vi "variantCtrlString.vi"(4 "isRequired (T)":bool=TRUE, 6 "menu in (get)":enum16{"get", "set"}(ring), 8 "error in":errorcluster, 9 "String Value":string, 10 "name in":string, 11 "Step in":variant) -> (0 "error out":errorcluster, 1 "String Value":string, 2 "isFound?":bool, 3 "Step out":variant)   [LabVIEW 2024]
uses:
  controls/typeEngErrorCodes.ctl
  controls/typeStepVarients.ctl
  controls/typeProcVarientName.ctl
panel:
  out "spreadsheet string":string
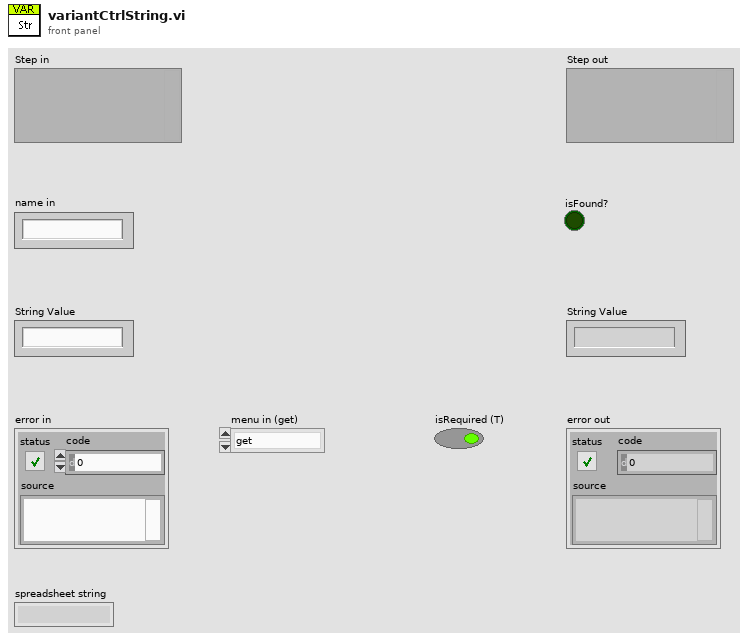
[diagram p1: front panel]
types:
  T1 = typedef "typeEngErrorCodes.ctl" = u16
  T2 = typedef "typeProcVarientName.ctl" = enum16{"procNameID", "procModuleID", "procPath", "procIsRunning", "procIndex", "procModule", "procRegisterNumeric", "procRegisterString", "procReport", "procReportPrev", "procCLK", "procStepPointer", "procType"}
  T3 = typedef "typeStepVarients.ctl" = enum16{"stepNameID", "stepFunction", "stepReport", "stepSetpoint", "stepPointer", "stepProcPointer", "stepIoPointer", "stepIoValue", "stepFilePointer", "stepMessage", "stepTimeString", "stepNumReg", "stepStrReg", "stepSeconds", "stepUnitDoseParams", "stepUnitIndex"}
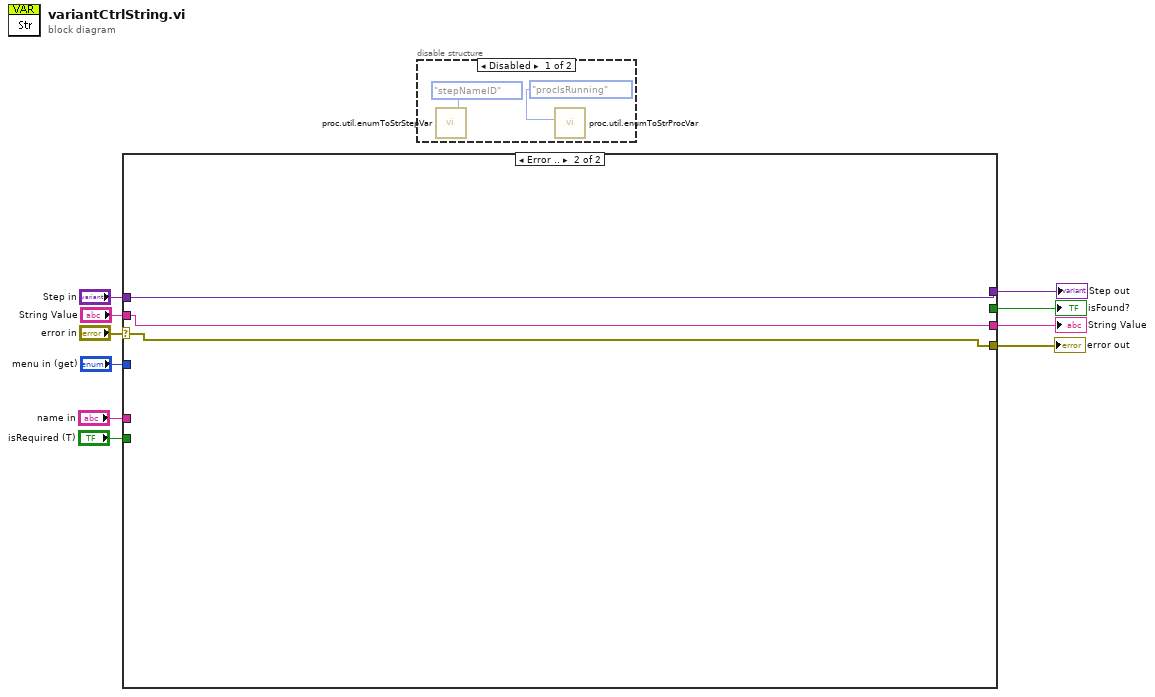
[diagram p0: block diagram]
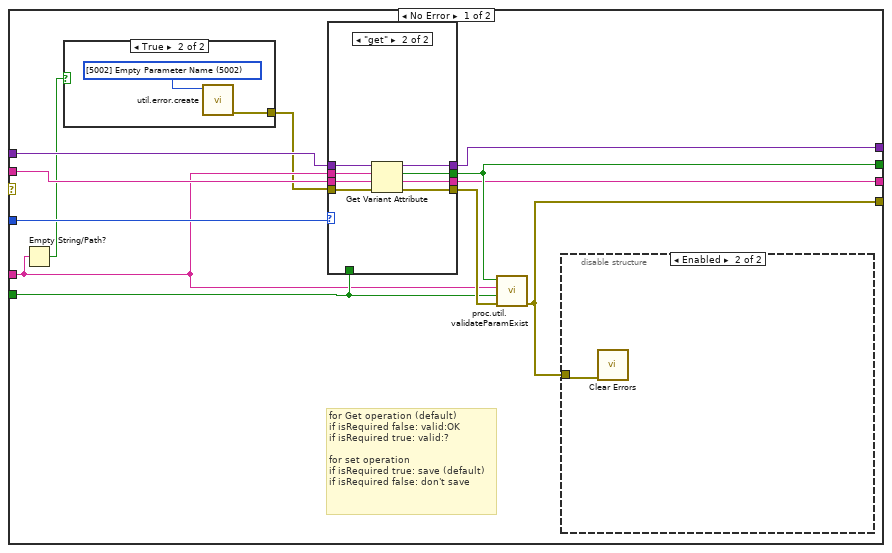
[diagram p2: hidden frame]
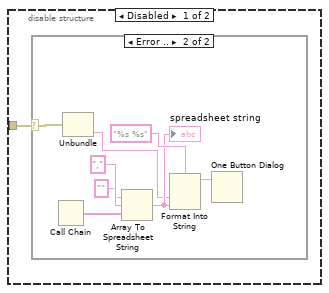
[diagram p4: hidden frame]
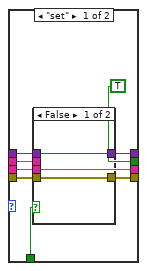
[diagram p6: hidden frame]
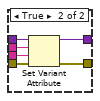
[diagram p7: hidden frame]
diagram:
  n1 = case shown="Error .." "error in" {
    selector: "error in" -> [_ w61]
    tunnel: "String Value" -> [w22 w59]
    tunnel: "Step in" -> [w21 w60]
    tunnel: [w15 w60] -> w8
    tunnel: "menu in (get)" -> [w20 _]
    tunnel: [w14 w59] -> w6
    tunnel: "isRequired (T)" -> [w16 _]
    tunnel: [w19 _] -> w4
    tunnel: "name in" -> [w13 _]
    tunnel: [w17 w61] -> w2
    frame No Error {
      # "for Get operation (default)\nif isRequired false: valid:OK\nif isRequired true: valid:?\n\nfor set operation\nif isRequired true: save (default)\nif isRequired false: don't save"
      n2 = Empty String/Path?(string/path=w13) -> (empty?=w12:bool)
      n3 = case shown="True" w12 {
        tunnel: [_ w23] -> w11
        frame False {
        }
        frame True {
          w24 = T1 5002 items=["[5000] Missing Function Arguments"=5000, "[5001] Incorrect Function Arguments"=5001, "[5002] Empty Parameter Name"=5002, "[5010] Not Found"=5010] ("Ring")
          n4 = call "util.error.create.vi"("Ring"=w24) -> ("error out"=w23:errorcluster)  [unwired: 9 in, 1 out]
        }
      }
      n5 = case shown="\"get\"" w20 {
        tunnel: w11 -> [w42 w58]
        tunnel: w22 -> [w37 w57]
        tunnel: w21 -> [w41 w56]
        tunnel: [w40 w55] -> w18
        tunnel: [TRUE w54] -> w19
        tunnel: [w39 w53] -> w15
        tunnel: w13 -> [w38 w52]
        tunnel: [w37 w51] -> w14
        tunnel: w16 -> [w35 _]
        frame "set" {
          n6 = case shown="False" w35 {
            tunnel: w42 -> [w43 w50]
            tunnel: w41 -> [w44 w49]
            tunnel: [w43 w48] -> w40
            tunnel: [w44 w47] -> w39
            tunnel: w38 -> [_ w46]
            tunnel: w37 -> [_ w45]
            frame False {
            }
            frame True {
              n7 = Set Variant Attribute(Variant=w49, name=w46, value=w45, error in=w50) -> (Variant out=w47:variant, error out=w48:errorcluster)  [unwired: 1 out]
            }
          }
        }
        frame "get" {
          n8 = Get Variant Attribute(Variant=w56, name=w52, default value (empty Variant)=w57, error in=w58) -> (duplicate Variant=w53:variant, found=w54:bool, value=w51:string, error out=w55:errorcluster)
        }
      }
      n9 = call "proc.util.validateParamExist.vi"("error in"=w18, "isRequired"=w16, "Param Label"=w13, "isFound"=w19) -> ("error out"=w17:errorcluster)  [unwired: 7 in]
      n10 = disable-structure shown="Enabled" {
        disable-tunnel: w17 -> [w25 w34]
        frame Disabled {
          n11 = case shown="Error .." w25 {
            selector: w25 -> [_ w33]
            frame No Error {
            }
            frame Error {
              n12 = Call Chain() -> (call chain=w32:string[])
              n13 = Unbundle(w33) -> ("source"=w26:string)  [unwired: 2 out]
              n14 = Array To Spreadsheet String(delimiter (Tab)=",", array=w32, 3:"" ("format string")) -> (spreadsheet string=w28:string)
              "spreadsheet string" <- w28
              n15 = Format Into String(format string="%s %s", w26, w28) -> (resulting string=w27:string)  [unwired: 2 in, 1 out]
              n16 = One Button Dialog(message=w27) -> ()  [unwired: 1 in, 1 out]
            }
          }
        }
        frame Enabled {
          n17 = call <vilib>:"Clear Errors.vi"("error in (no error)"=w34) -> ()  [unwired: 5 in, 2 out]
        }
      }
    }
    frame Error {
    }
  }
  "error out" <- w2
  "isFound?" <- w4
  "Step out" <- w8
  "String Value" <- w6
  n18 = disable-structure shown="Disabled" {
    frame Disabled {
      n19 = call "proc.util.enumToStrStepVar.vi"("Step var"=typeStepVarients."stepNameID") -> ()  [unwired: 10 in, 1 out]
      n20 = call "proc.util.enumToStrProcVar.vi"("Proc var"=typeProcVarientName."procIsRunning") -> ()  [unwired: 10 in, 1 out]
    }
    frame Enabled {
    }
  }
